vi "Main - Intilization RT.vi"(8 "Error In":errorcluster) -> (0 "Error Out":errorcluster)   [LabVIEW 2020]
uses:
  Control/FGV State.ctl
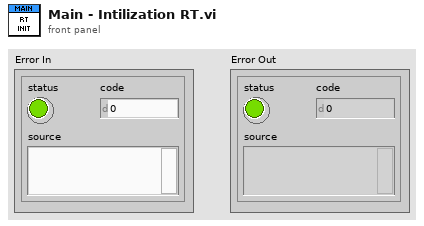
[diagram p1: front panel]
types:
  T1 = enum16{"Init Path", "Create Config File", "Init Variables", "Module Info", "Close"}
  T2 = typedef "FGV State.ctl" = enum16{"Write", "Read"}
  T3 = typedef "Modules Info.ctl" = cluster{"Product Name":string, "Product Type ":string, "I/Os":tag[]}
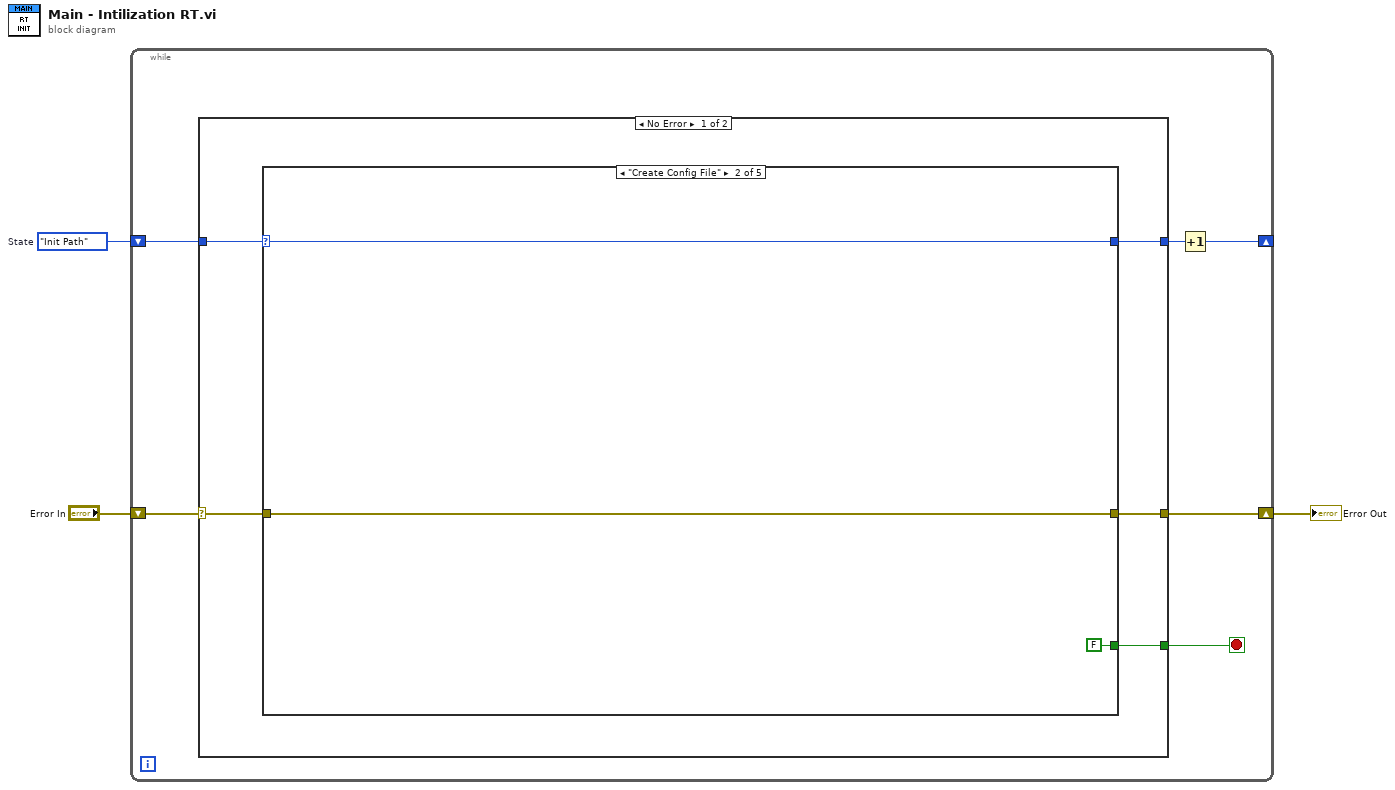
[diagram p0: block diagram]
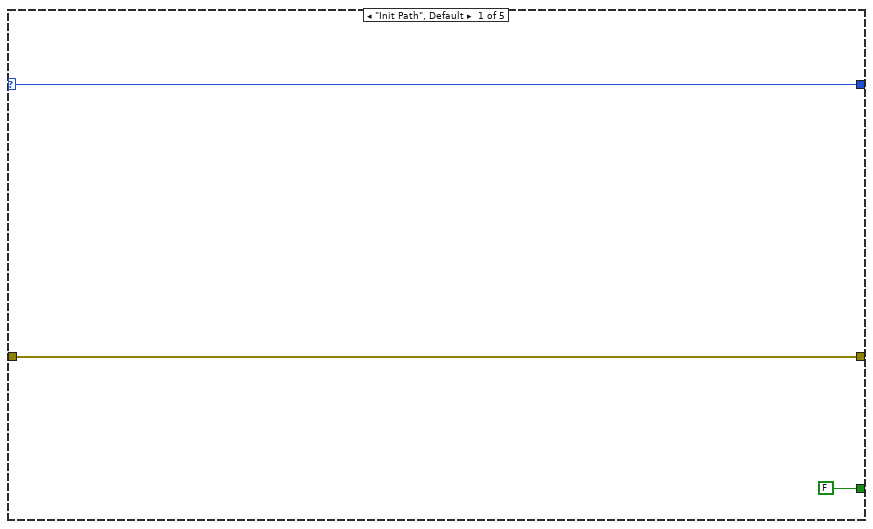
[diagram p2: hidden frame]
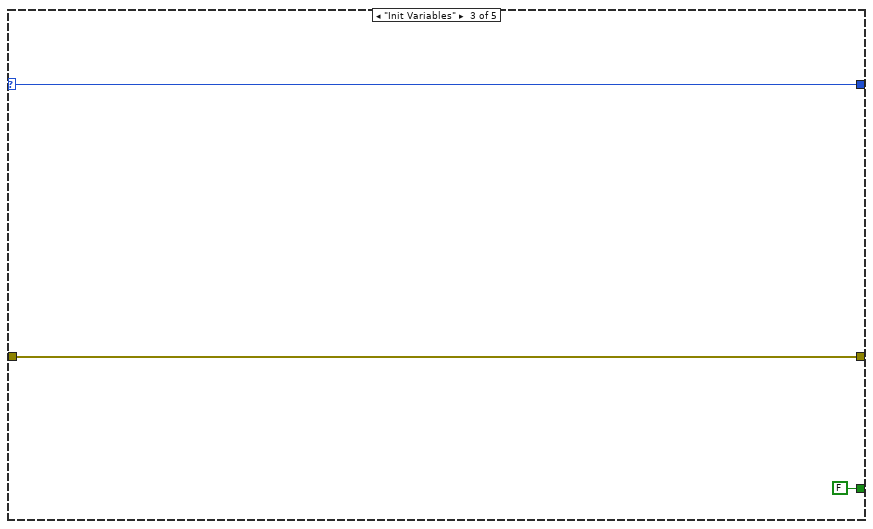
[diagram p3: hidden frame]
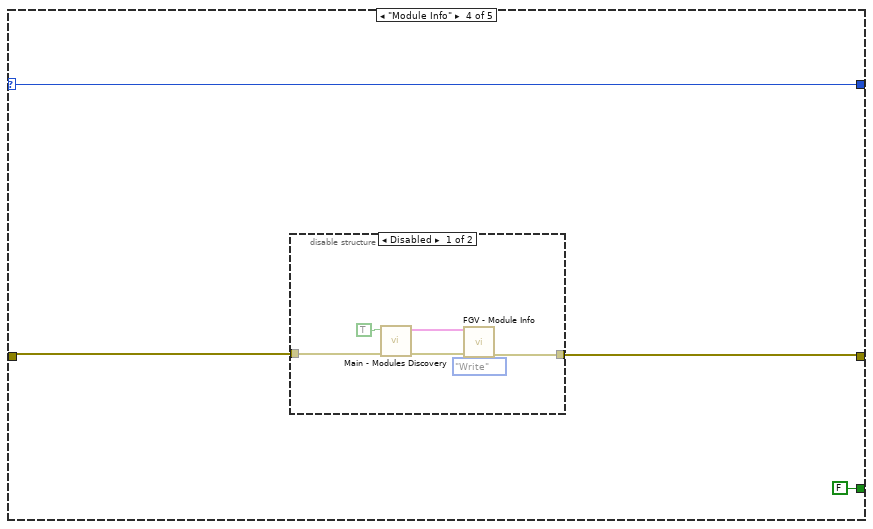
[diagram p4: hidden frame]
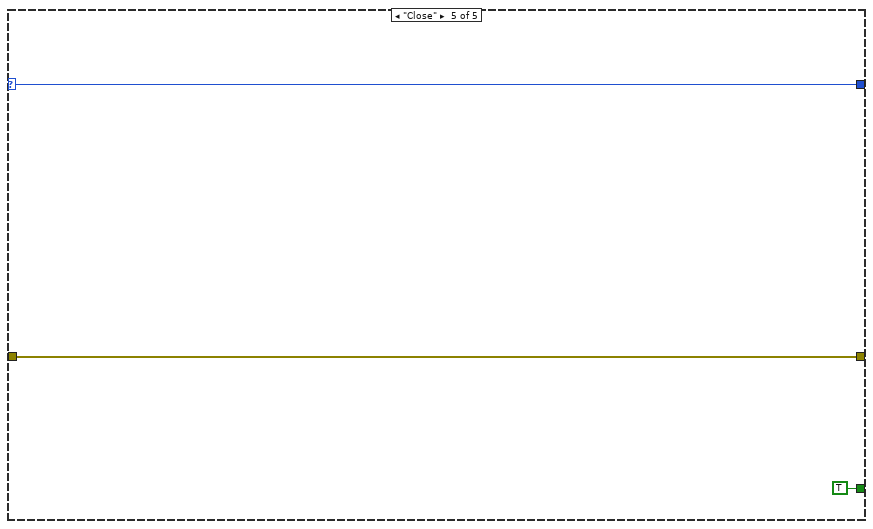
[diagram p6: hidden frame]
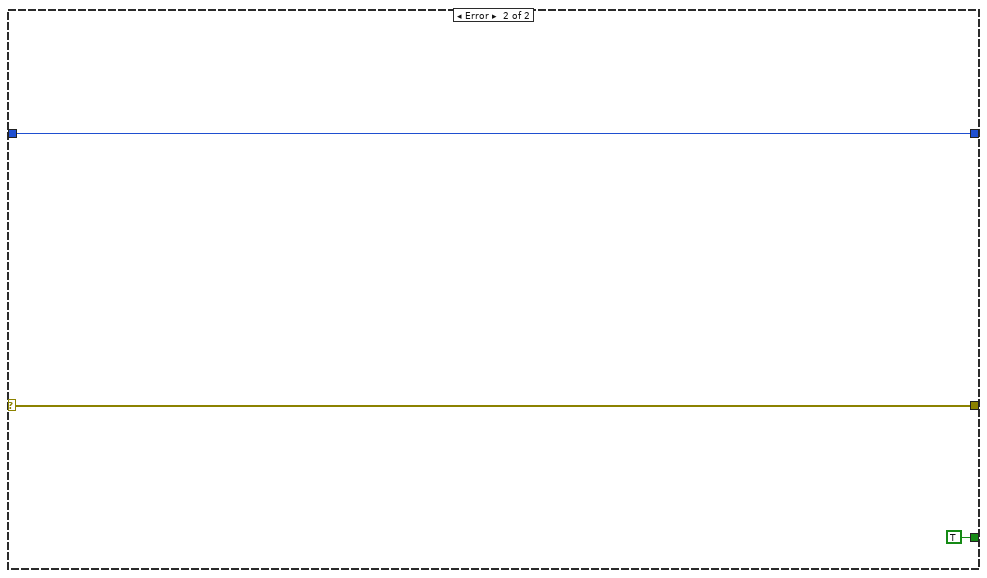
[diagram p7: hidden frame]
diagram:
  w1 = T1."Init Path"  # State
  n1 = while {
    shift-right: [w8] -> w2
    shift-left: "Error In" -> [w9]
    shift-right: [w5] -> _
    shift-left: w1 -> [w7]
    stop <- w4 stop-if-true
    n2 = case shown="No Error" w9 {
      selector: w9 -> [w13 w39]
      tunnel: [w14 w39] -> w8
      tunnel: w7 -> [w12 w38]
      tunnel: [w11 w38] -> w6
      tunnel: [w10 TRUE] -> w4
      frame No Error {
        n3 = case shown="\"Create Config File\"" w12 {
          selector: w12 -> [w17 w20 w23 w24 w35]
          tunnel: [w15 w18 w21 w26 w36] -> w14
          tunnel: w13 -> [w15 w18 w21 w27 w36]
          tunnel: [w17 w20 w23 w24 w35] -> w11
          tunnel: [FALSE FALSE FALSE FALSE TRUE] -> w10
          frame "Init Path", Default {
          }
          frame "Create Config File" {
          }
          frame "Init Variables" {
          }
          frame "Module Info" {
            n4 = disable-structure shown="Disabled" {
              disable-tunnel: w27 -> [w32 _]
              disable-tunnel: [w31 _] -> w26
              frame Disabled {
                n5 = call "Main - Modules Discovery.vi"("Error In"=w32, "Allow Simulated Device? (F)"=TRUE) -> ("Error Out"=w33:errorcluster, "Modules Info Array"=w29:T3[])  [unwired: 8 in]
                n6 = call "FGV - Module Info.vi"("FGV State"=FGV_State."Write", "Error In"=w33, "Module Info"=w29) -> ("Error Out"=w31:errorcluster)  [unwired: 7 in, 1 out]
              }
              frame Enabled {
              }
            }
          }
          frame "Close" {
          }
        }
      }
      frame Error {
      }
    }
    n7 = Increment(x=w6) -> (x+1=w5:T1)
  }
  "Error Out" <- w2
